vi "Simplify error message.vi"(8 "error in (no error)":errorcluster, 10 "Source":string, 11 "Code":i32) -> (0 "error out":errorcluster, 3 "String":string)   [LabVIEW 2017, in "File IO.lvlib"]
uses:
  File IO.lvlib
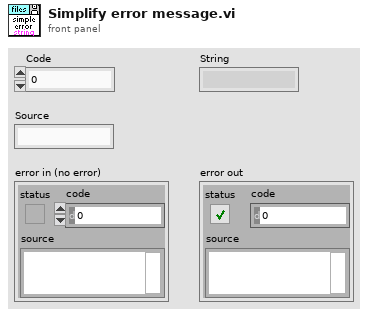
[diagram p1: front panel]
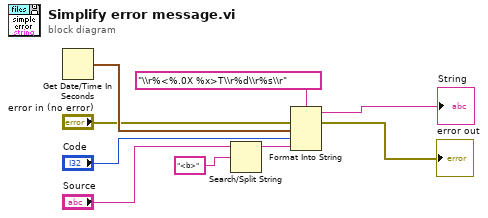
[diagram p0: block diagram]
diagram:
  n1 = Get Date/Time In Seconds() -> (seconds since 1Jan1904=w9:timestamp)
  n2 = Search/Split String(string="Source", search string/char (-)="<b>") -> (substring before match=w7:string)  [unwired: 1 in, 2 out]
  n3 = Format Into String(format string="\\r%<%.0X %x>T\\r%d\\r%s\\r", error in="error in (no error)", w9, "Code", w7) -> (resulting string=→"String":string, error out=→"error out":errorcluster)  [unwired: 1 in]
